vi "Create Set of Rocks.vi"(11 "Grid In":bool[][](array[boolean])) -> (3 "Rock Positions":cluster{i32, i32}[](array[cluster]))   [LabVIEW 2021]
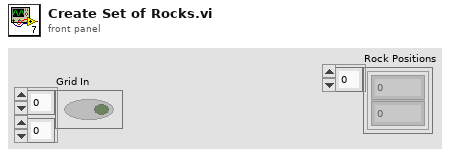
[diagram p1: front panel]
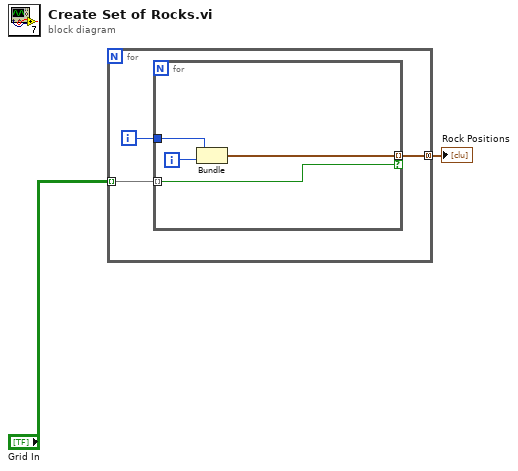
[diagram p0: block diagram]
diagram:
  n1 = for {
    tunnel: "Grid In" -> [w5] mode=indexing
    tunnel: [w3] -> w1 mode=concatenating
    i -> [w4]
    n2 = for {
      tunnel: w5 -> [w6] mode=indexing
      tunnel: w4 -> [w8]
      tunnel: [w7] -> w3 mode=indexing if=w6
      i -> [w9]
      n3 = Bundle(w8, w9) -> (w7:cluster{i32, i32})  [unwired: 1 in]
    }
  }
  "Rock Positions" <- w1
